vi "Read msec between samples.vi"(4 "Error In":errorcluster, 7 "Set Acquisition Rate in":refnum<class "Remote Access Commands_Set Acquisition Rate.lvclass">) -> (0 "Error Out":errorcluster, 2 "msec between samples":i32, 3 "Set Acquisition Rate out":refnum<class "Remote Access Commands_Set Acquisition Rate.lvclass">)   [LabVIEW 2015, in "Startup Processes.lvlib" / "Remote Access Commands_Set Acquisition Rate.lvclass"]
uses:
  Remote Access Commands_Set Acquisition Rate.lvclass
  Remote Access Commands_Set Acquisition Rate.lvclass/Remote Access Commands_Set Acquisition Rate.ctl
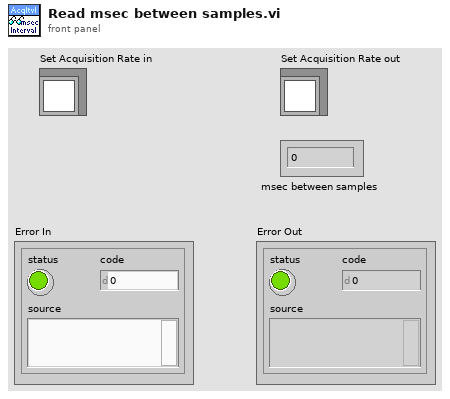
[diagram p1: front panel]
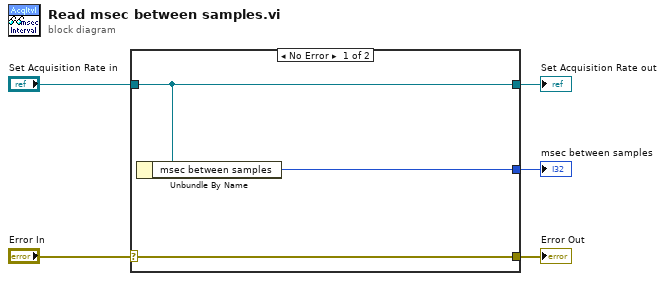
[diagram p0: block diagram]
diagram:
  n1 = case shown="No Error" "Error In" {
    selector: "Error In" -> [w8 w9]
    tunnel: [w8 w9] -> w4
    tunnel: [w7 w10] -> w2
    tunnel: "Set Acquisition Rate in" -> [w7 w10]
    tunnel: [w6 _] -> w1
    frame No Error {
      n2 = Unbundle By Name(w7) -> ("msec between samples"=w6:i32)
    }
    frame Error {
    }
  }
  "Error Out" <- w4
  "Set Acquisition Rate out" <- w2
  "msec between samples" <- w1
